vi "WebSocket Connection State Callback.vi"(7 "Owner":refnum<class>, 8 "error in (no error)":errorcluster, 9 "Context":variant, 10 "Connection State":T1, 11 "Connection":refnum<class "Connection.lvclass">) -> (0 "error out":errorcluster)   [LabVIEW 2020, in "GodotLV.lvlib" / "GodotServer.lvclass"]
uses:
  GodotServer.lvclass
  lv-stream-websocket/Stream-Websocket/WebsocketStream/WebsocketStream.lvclass
  lv-stream/stream/Connection/Connection.lvclass
  lv-stream/stream/Connection State.ctl
  lv-stream/stream/Stream.lvlib
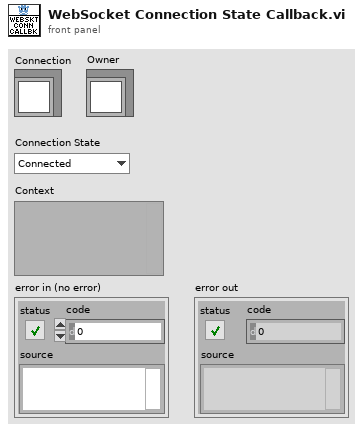
[diagram p1: front panel]
types:
  T1 = typedef "Stream.lvlib/Connection State.ctl" = enum16{"Connected", "Disconnected"}
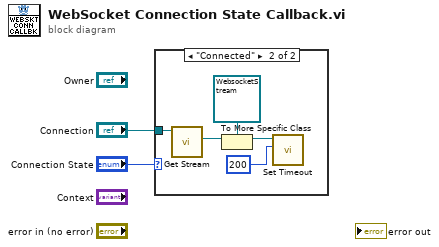
[diagram p0: block diagram]
diagram:
  n1 = case shown="\"Connected\"" "Connection State" {
    tunnel: "Connection" -> [_ w7]
    frame "Disconnected" {
    }
    frame "Connected" {
      n2 = call-dynamic "Get Stream.vi"("Connection in"=w7) -> ("Stream"=w6:refnum<class "Stream.lvclass">)  [unwired: 8 in, 2 out]
      n3 = To More Specific Class(target class=refnum<class "WebsocketStream.lvclass"> refnum ("Stream-Websocket:WebsocketStream"), reference=w6) -> (specific class reference=w4:refnum<class "WebsocketStream.lvclass">)  [unwired: 1 in, 1 out]
      n4 = call "Set Timeout.vi"("Timeout ms"=200, "WebsocketStream in"=w4) -> ()  [unwired: 8 in, 2 out]
    }
  }
